vi "fpga_8ch_Timestamping_BaselineCh_ov.vi"(0 "Main clock":u32, 1 "Scheduler":u8, 2 "Baseline Ch":u8, 3 "Signal IN":T1, 4 "overflow":bool) -> (5 "Data available":T1, 6 "Timestamp bundle":T2)   [LabVIEW 2011]
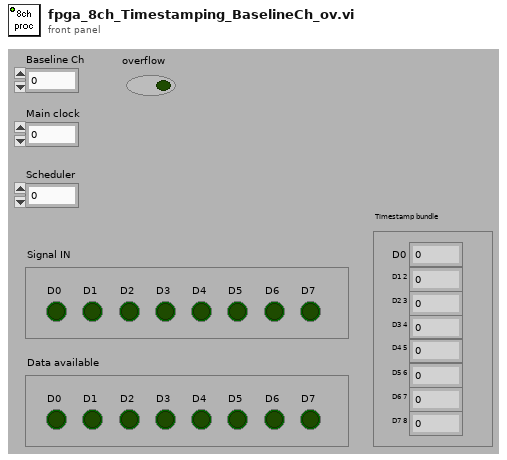
[diagram p1: front panel]
types:
  T1 = cluster{"D0":bool, "D1":bool, "D2":bool, "D3":bool, "D4":bool, "D5":bool, "D6":bool, "D7":bool}
  T2 = cluster{"D0":u32, "D1 2":u32, "D2 3":u32, "D3 4":u32, "D4 5":u32, "D5 6":u32, "D6 7":u32, "D7 8":u32}
  T3 = cluster{"Data Available":bool, "Data Available":bool, "Data Available":bool, "Data Available":bool, "Data Available":bool, "Data Available":bool, "Data Available":bool, "Data Available":bool}
  T4 = cluster{"32 bit Output":u32, "32 bit Output":u32, "32 bit Output":u32, "32 bit Output":u32, "32 bit Output":u32, "32 bit Output":u32, "32 bit Output":u32, "32 bit Output":u32}
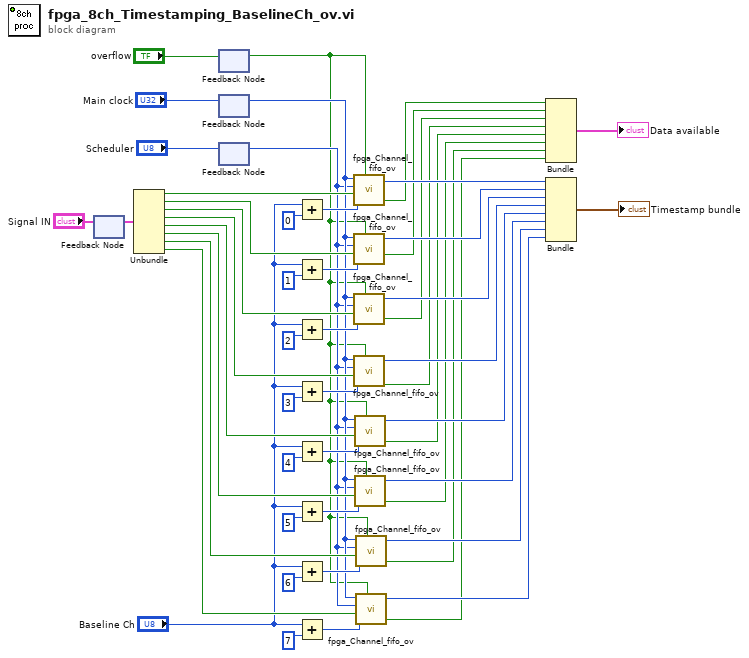
[diagram p0: block diagram]
diagram:
  n1 = feedback-in #1("Signal IN") -> ()
  n2 = feedback #1() -> (w3:T1)  [unwired: 1 in]
  n3 = Unbundle(w3) -> ("D0"=w50:bool, "D1"=w49:bool, "D2"=w48:bool, "D3"=w47:bool, "D4"=w46:bool, "D5"=w45:bool, "D6"=w44:bool, "D7"=w43:bool)
  n4 = feedback #2() -> (w1:bool)  [unwired: 1 in]
  n5 = feedback-in #2("overflow") -> ()
  n6 = feedback-in #3("Main clock") -> ()
  n7 = feedback #3() -> (w6:u32)  [unwired: 1 in]
  n8 = feedback #4() -> (w4:u8)  [unwired: 1 in]
  n9 = feedback-in #4("Scheduler") -> ()
  n10 = Add(x="Baseline Ch", y=u8 0 ("ID")) -> (x+y=w23:u8)
  n11 = Add(x="Baseline Ch", y=u8 1 ("ID")) -> (x+y=w10:u8)
  n12 = Add(x="Baseline Ch", y=u8 2 ("ID")) -> (x+y=w11:u8)
  n13 = Add(x="Baseline Ch", y=u8 3 ("ID")) -> (x+y=w8:u8)
  n14 = Add(x="Baseline Ch", y=u8 4 ("ID")) -> (x+y=w12:u8)
  n15 = Add(x="Baseline Ch", y=u8 5 ("ID")) -> (x+y=w13:u8)
  n16 = Add(x="Baseline Ch", y=u8 6 ("ID")) -> (x+y=w14:u8)
  n17 = Add(x="Baseline Ch", y=u8 7 ("ID")) -> (x+y=w15:u8)
  n18 = call "fpga_Channel_fifo_ov.vi"("Main clock"=w6, "Scheduler"=w4, "Signal IN"=w50, "ID"=w23, "overflow"=w1) -> ("32 bit Output"=w42:u32, "Data Available"=w33:bool)  [unwired: 1 out]
  n19 = call "fpga_Channel_fifo_ov.vi"("Main clock"=w6, "Scheduler"=w4, "Signal IN"=w49, "ID"=w10, "overflow"=w1) -> ("32 bit Output"=w41:u32, "Data Available"=w32:bool)  [unwired: 1 out]
  n20 = call "fpga_Channel_fifo_ov.vi"("Main clock"=w6, "Scheduler"=w4, "Signal IN"=w48, "ID"=w11, "overflow"=w1) -> ("32 bit Output"=w40:u32, "Data Available"=w31:bool)  [unwired: 1 out]
  n21 = call "fpga_Channel_fifo_ov.vi"("Main clock"=w6, "Scheduler"=w4, "Signal IN"=w47, "ID"=w8, "overflow"=w1) -> ("32 bit Output"=w39:u32, "Data Available"=w30:bool)  [unwired: 1 out]
  n22 = call "fpga_Channel_fifo_ov.vi"("Main clock"=w6, "Scheduler"=w4, "Signal IN"=w46, "ID"=w12, "overflow"=w1) -> ("32 bit Output"=w38:u32, "Data Available"=w29:bool)  [unwired: 1 out]
  n23 = call "fpga_Channel_fifo_ov.vi"("Main clock"=w6, "Scheduler"=w4, "Signal IN"=w45, "ID"=w13, "overflow"=w1) -> ("32 bit Output"=w37:u32, "Data Available"=w28:bool)  [unwired: 1 out]
  n24 = call "fpga_Channel_fifo_ov.vi"("Main clock"=w6, "Scheduler"=w4, "Signal IN"=w44, "ID"=w14, "overflow"=w1) -> ("32 bit Output"=w36:u32, "Data Available"=w27:bool)  [unwired: 1 out]
  n25 = call "fpga_Channel_fifo_ov.vi"("Main clock"=w6, "Scheduler"=w4, "Signal IN"=w43, "ID"=w15, "overflow"=w1) -> ("32 bit Output"=w35:u32, "Data Available"=w26:bool)  [unwired: 1 out]
  n26 = Bundle("Data Available"=w33, "Data Available"=w32, "Data Available"=w31, "Data Available"=w30, "Data Available"=w29, "Data Available"=w28, "Data Available"=w27, "Data Available"=w26) -> (→"Data available":T3)  [unwired: 1 in]
  n27 = Bundle("32 bit Output"=w42, "32 bit Output"=w41, "32 bit Output"=w40, "32 bit Output"=w39, "32 bit Output"=w38, "32 bit Output"=w37, "32 bit Output"=w36, "32 bit Output"=w35) -> (→"Timestamp bundle":T4)  [unwired: 1 in]
